vi "习4.5.vi"() -> ()   [LabVIEW 2017]
panel:
  out "数值":dbl
  in  "指定值":dbl
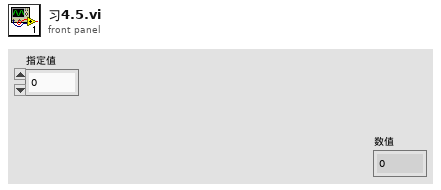
[diagram p1: front panel]
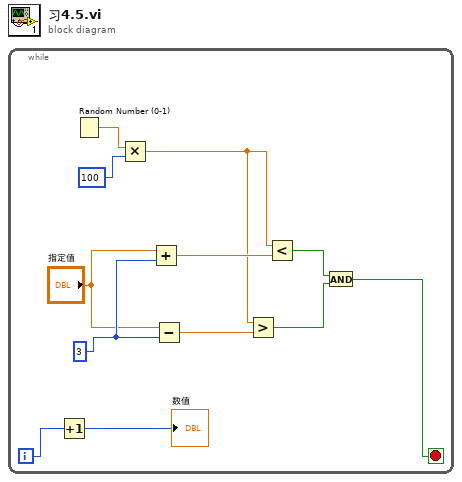
[diagram p0: block diagram]
diagram:
  n1 = while {
    i -> [w2]
    stop <- w3 stop-if-true
    w10 = 3
    n2 = Increment(x=w2) -> (x+1=→"数值":i32)
    n3 = Random Number (0-1)() -> (number: 0 to 1=w12:dbl)
    n4 = Multiply(x=w12, y=100) -> (x*y=w6:dbl)
    n5 = Add(x="指定值", y=w10) -> (x+y=w8:dbl)
    n6 = Subtract(x="指定值", y=w10) -> (x-y=w7:dbl)
    n7 = Greater?(x=w6, y=w7) -> (0:w4:bool)
    n8 = Less?(x=w6, y=w8) -> (x < y?=w5:bool)
    n9 = And(x=w5, y=w4) -> (x .and. y?=w3:bool)
  }
